vi "Byte69_82_temperature_conversion (SubVI).vi"(1 "Numeric":u16) -> (0 "Control Card Temperature value":dbl)   [LabVIEW 2024]
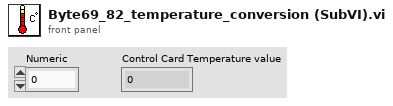
[diagram p1: front panel]
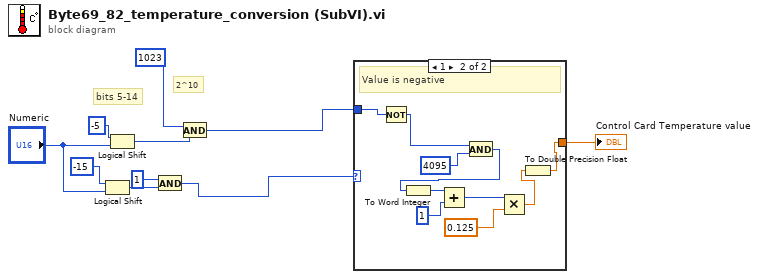
[diagram p0: block diagram]
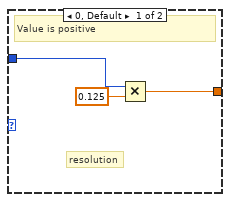
[diagram p2: hidden frame]
diagram:
  # "2^10"
  # "bits 5-14"
  n1 = Logical Shift(y=i16 -15, x="Numeric") -> (x << y=w5:u16)
  n2 = Logical Shift(y=i16 -5, x="Numeric") -> (x << y=w2:u16)
  n3 = And(x=u16 1, y=w5) -> (x .and. y?=w7:u16)
  n4 = And(x=u16 1023, y=w2) -> (x .and. y?=w8:u16)
  n5 = case shown="1" w7 {
    tunnel: w8 -> [w13 w20]
    tunnel: [w11 w18] -> w9
    frame 0, Default {
      # "resolution"
      # "Value is positive"
      n6 = Multiply(x=w13, y=0.125) -> (x*y=w11:dbl)
    }
    frame 1 {
      # "Value is negative"
      n7 = Not(x=w20) -> (.not. x?=w17:u16)
      n8 = And(x=w17, y=u16 4095) -> (x .and. y?=w15:u16)
      n9 = To Word Integer(number=w15) -> (16bit integer=w14:i16)
      n10 = Add(x=w14, y=i16 1) -> (x+y=w22:i16)
      n11 = Multiply(x=w22, y=0.125) -> (x*y=w19:dbl)
      n12 = To Double Precision Float(number=w19) -> (double precision float=w18:dbl)
    }
  }
  "Control Card Temperature value" <- w9
